vi "getValue.vi"(8 "error in (no error)":errorcluster, 11 "tBSONBinary in":refnum<class "tBSONBinary.lvclass">) -> (0 "error out":errorcluster, 2 "Value":u8[](array[numeric]), 3 "tBSONBinary out":refnum<class "tBSONBinary.lvclass">)   [LabVIEW 2013, in "BSON.lvlib" / "tBSONBinary.lvclass"]
uses:
  tBSONBinary.lvclass
  tBSONBinary.lvclass/tBSONBinary.ctl
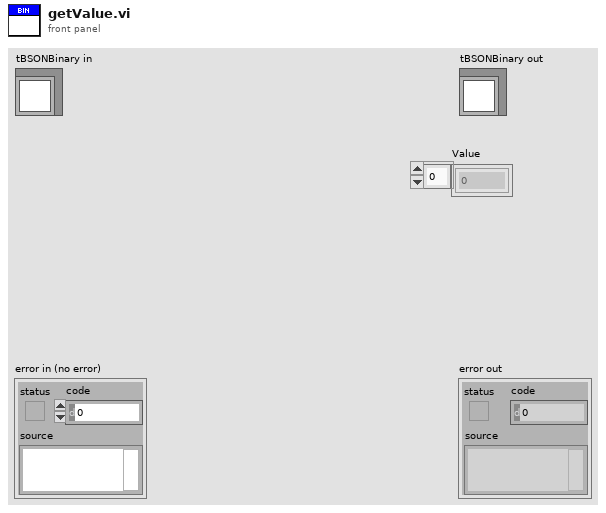
[diagram p1: front panel]
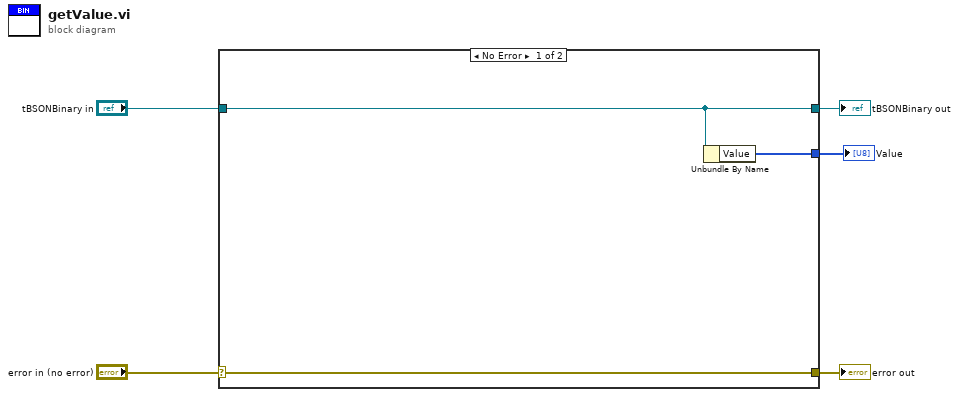
[diagram p0: block diagram]
diagram:
  n1 = case shown="No Error" "error in (no error)" {
    selector: "error in (no error)" -> [w8 w10]
    tunnel: [w8 w10] -> w4
    tunnel: [w7 w9] -> w2
    tunnel: "tBSONBinary in" -> [w7 w9]
    tunnel: [w6 _] -> w1
    frame No Error {
      n2 = Unbundle By Name(w7) -> ("Value"=w6:u8[])
    }
    frame Error {
    }
  }
  "error out" <- w4
  "tBSONBinary out" <- w2
  "Value" <- w1
